vi "DataReady Event Callback.vi"(4 "notifier out":refnum<notifier>, 6 "CtlRef":refnum<k7>, 7 "Event common data":cluster{"Source":i32, "Type":u32, "Time":u32}) -> ()   [LabVIEW 2009]
doc: "Description:\nThis is a callback VI that gets called when the ActiveX fires the DataReady event to notify the client application that a new packet of measurements has been received. The main VI then calls the GetData method to gather the data packet from the ActiveX, afterwards parsing and processing the received data.\n\nInputs: \nEvent common data: Source of the event, type, and timestamp\nCtlRef: Wire the ActiveX refnum to this\nNotifier Out: Event to fire to the rest of the LabVIEW application\n\nOutputs:\nNone\n\nPossible Error Codes\nNone"
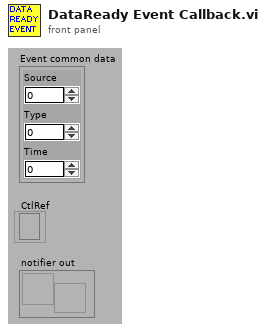
[diagram p1: front panel]
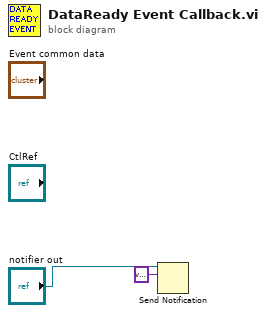
[diagram p0: block diagram]
diagram:
  n1 = Send Notification(notification=variant, notifier="notifier out") -> ()  [unwired: 1 in, 2 out]
